vi "New Figure Object.vi"(8 "error in (no error)":errorcluster, 11 "xwpfRun.Figure in":refnum<class "xwpfRun.Figure.lvclass">) -> (0 "error out":errorcluster, 3 "xwpfRun.Figure out":refnum<class "xwpfRun.Figure.lvclass">)   [LabVIEW 2017, in "Word_Specific.lvlib" / "xwpfRun.Figure.lvclass"]
uses:
  xwpfRun.Figure.lvclass
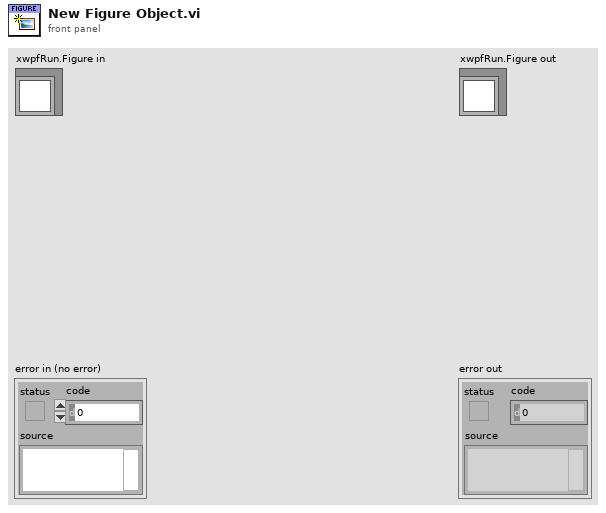
[diagram p1: front panel]
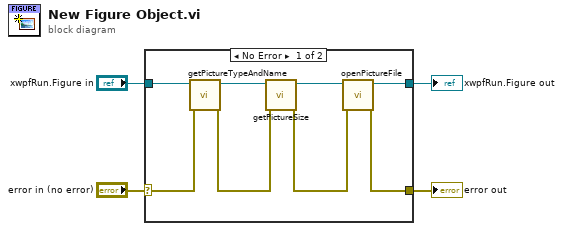
[diagram p0: block diagram]
diagram:
  n1 = case shown="No Error" "error in (no error)" {
    selector: "error in (no error)" -> [w12 w14]
    tunnel: [w9 w14] -> w3
    tunnel: [w5 w13] -> w1
    tunnel: "xwpfRun.Figure in" -> [w8 w13]
    frame No Error {
      n2 = call "getPictureTypeAndName.vi"("error in (no error)"=w12, "xwpfRun.Figure in"=w8) -> ("error out"=w10:errorcluster, "xwpfRun.Figure out"=w11:refnum<class "xwpfRun.Figure.lvclass">)  [unwired: 8 in]
      n3 = call "getPictureSize.vi"("error in (no error)"=w10, "xwpfRun.Figure in"=w11) -> ("error out"=w6:errorcluster, "xwpfRun.Figure out"=w7:refnum<class "xwpfRun.Figure.lvclass">)  [unwired: 8 in]
      n4 = call "openPictureFile.vi"("error in (no error)"=w6, "xwpfRun.Figure in"=w7) -> ("error out"=w9:errorcluster, "xwpfRun.Figure out"=w5:refnum<class "xwpfRun.Figure.lvclass">)  [unwired: 8 in]
    }
    frame Error {
    }
  }
  "error out" <- w3
  "xwpfRun.Figure out" <- w1
